vi "testing.vi"(7 "httpRequestID":u32) -> ()   [LabVIEW 2011]
doc: "This VI is a state machine that can be ran from a Browser."
uses:
  server/database/Users/User Record.ctl
  <vilib>/wsapi/NI_WebServices.lvlib
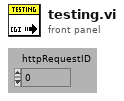
[diagram p1: front panel]
types:
  T1 = typedef "User Record.ctl" = cluster{"ixUser":i32, "sxUsername":string, "sLastName":string, "sFirstName":string, "sEmail":string, "sPassword":string, "tLoginTime":timestamp, "sLoginComputer":string, "fAdministrator":bool, "fRunSequences":bool, "fModifySequences":bool, "fRunScenarios":bool, "fModifyScenarios":bool, "fModifyTemplates":bool, "fModifyUsers":bool, "fModifyStations":bool, "fModifyFields":bool}
  T2 = typedef "Connection Refnum.ctl" = cluster{"Environment Handle":i32, "Connection Handle":i32}
  T3 = typedef "Keyed Array.ctl" = cluster{"keys":string[], "values":string[]}
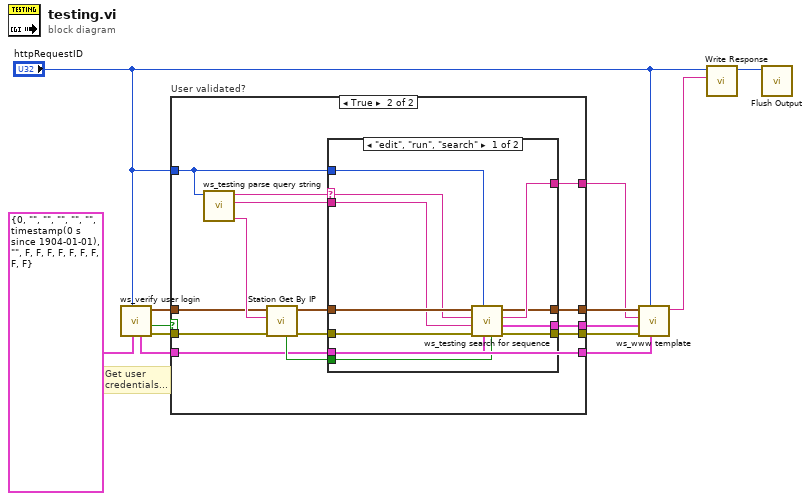
[diagram p0: block diagram]
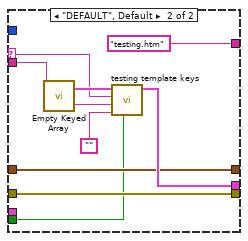
[diagram p3: hidden frame]
diagram:
  # "Get user \ncredentials..."
  n1 = call "ws_verify user login.vi"("Required Permisions"=T1 {"ixUser"=0, "sxUsername"="", "sLastName"="", "sFirstName"="", "sEmail"="", "sPassword"="", "tLoginTime"=timestamp(0 s since 1904-01-01), "sLoginComputer"="", "fAdministrator"=FALSE, "fRunSequences"=FALSE, "fModifySequences"=FALSE, "fRunScenarios"=FALSE, "fModifyScenarios"=FALSE, "fModifyTemplates"=FALSE, "fModifyUsers"=FALSE, "fModifyStations"=FALSE, "fModifyFields"=FALSE} ("User Record"), "httpRequestID"="httpRequestID") -> ("error out"=w13:errorcluster, "User Verified\nand Spartan\nAuthorized?"=w12:bool, "DB Connection Ref"=w11:T2, "User"=w10:T1)  [unwired: 6 in]
  n2 = case "User validated?" shown="True" w12 {
    tunnel: w10 -> [w15 w19]
    tunnel: w11 -> [w14 w22]
    tunnel: w13 -> [w16 w21]
    tunnel: [w16 w24] -> w8
    tunnel: [w14 w23] -> w7
    tunnel: [_ w18] -> w3
    tunnel: [w15 w19] -> w2
    tunnel: [_ w20] -> w4
    tunnel: "httpRequestID" -> [_ w17]
    frame False {
    }
    frame True {
      n3 = call "ws_testing parse query string.vi"("httpRequestID"=w17) -> ("Client Address"=w26:string, "TestSeqId"=w29:string, "Action"=w30:string)  [unwired: 8 in]
      n4 = call "Station Get By IP.vi"("error in (no error)"=w21, "IP or Name (\"\")"=w26, "Connection Refnum"=w22) -> ("error out"=w27:errorcluster, "Connection Refnum"=w28:T2, "Data Present?"=w25:bool)  [unwired: 6 out]
      n5 = case shown="\"edit\", \"run\", \"search\"" w30 {
        selector: w30 -> [w34 w47]
        tunnel: [w39 "testing.htm" ("Template (\"\")")] -> w18
        tunnel: [w38 w45] -> w24
        tunnel: w27 -> [w41 w45]
        tunnel: w19 -> [w35 _]
        tunnel: w28 -> [w37 w46]
        tunnel: [w36 w46] -> w23
        tunnel: [w40 w48] -> w20
        tunnel: w29 -> [w33 w43]
        tunnel: w25 -> [w32 w44]
        tunnel: w17 -> [w31 _]
        frame "edit", "run", "search" {
          n6 = call "ws_testing search for sequence.vi"("Test Station? (f)"=w32, "User"=w35, "httpRequestID"=w31, "error in (no error)"=w41, "TestSeqId (\"\")"=w33, "Action (\"Search\")"=w34, "Connection Refnum"=w37) -> ("error out"=w38:errorcluster, "Template Keys"=w40:T3, "Template"=w39:string, "Connection Refnum"=w36:T2)  [unwired: 1 in]
        }
        frame "DEFAULT", Default {
          n7 = call "Empty Keyed Array.vi"() -> ("empty keyed array"=w49:T3)  [unwired: 3 out]
          n8 = call "testing template keys.vi"("Test Station? (f)"=w44, "$$SEQLIST$$ (\"\")"="", "$$SEQID$$ (\"\")"=w43, "$$MODE$$ (\"\")"=w47, "Keys In"=w49) -> ("Keys Out"=w48:T3)  [unwired: 1 in, 5 out]
        }
      }
    }
  }
  n9 = call "ws_www template.vi"("User"=w2, "httpRequestID"="httpRequestID", "error in (no error)"=w8, "Template Keys (empty)"=w4, "Template (\"\")"=w3, "DB Connection Ref"=w7) -> ("HTTP Template Content"=w6:string)  [unwired: 5 in]
  n10 = call <vilib>:"Write Response.vi"("response string"=w6, "httpRequestID"="httpRequestID") -> ("httpRequestID out"=w5:u32)  [unwired: 8 in, 1 out]
  n11 = call <vilib>:"Flush Output.vi"("httpRequestID"=w5) -> ()  [unwired: 9 in, 2 out]
